vi "Msg To.vi"(10 "Error":errorcluster) -> (3 "Merge Error Msg Strategy out":refnum<class "Merge Error Msg Strategy.lvclass">)   [LabVIEW 2021, in "jettl.lvlib" / "Merge Error.lvlib" / "Merge Error Msg Strategy.lvclass"]
uses:
  Merge Error Msg Strategy.lvclass
  Merge Error Msg Strategy.lvclass/Merge Error Msg Strategy.ctl
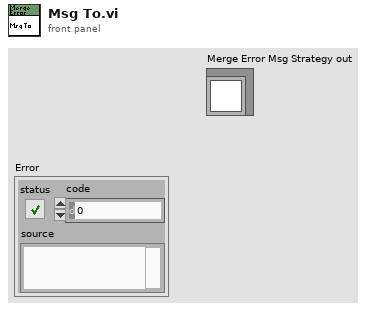
[diagram p1: front panel]
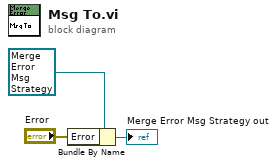
[diagram p0: block diagram]
diagram:
  n1 = Bundle By Name(cluster=refnum<class "Merge Error Msg Strategy.lvclass"> refnum ("Merge Error Msg Strategy out"), "Error"="Error") -> (→"Merge Error Msg Strategy out":refnum<class "Merge Error Msg Strategy.lvclass">)
